vi "Rotate_Blade.vi"(7 "Activate Rotation?":bool, 8 "error in":errorcluster, 9 "Axis":cluster{"X":sgl, "Y":sgl, "Z":sgl}, 10 "angle":sgl, 11 "Scene Object In":refnum<vi>) -> (0 "error out":errorcluster, 3 "Scene Object Out":refnum<vi>)   [LabVIEW 2019]
uses:
  <vilib>/picture/3D Picture Control/NI_3D Picture Control.lvlib
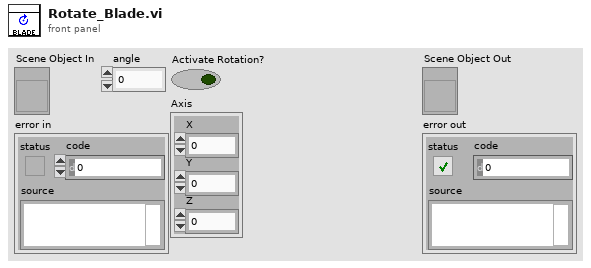
[diagram p1: front panel]
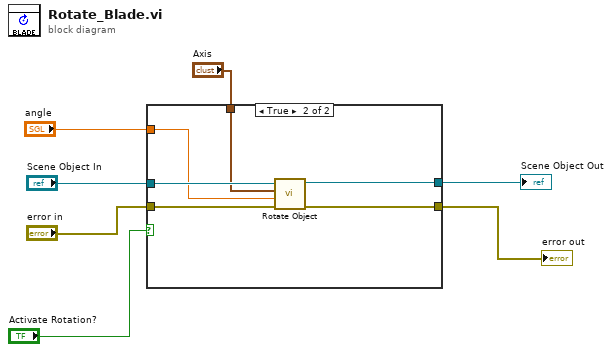
[diagram p0: block diagram]
diagram:
  n1 = case shown="True" "Activate Rotation?" {
    tunnel: [w9 w15] -> w7
    tunnel: "Scene Object In" -> [w9 w14]
    tunnel: "error in" -> [w8 w13]
    tunnel: [w8 w12] -> w4
    tunnel: "angle" -> [_ w11]
    tunnel: "Axis" -> [_ w10]
    frame False {
    }
    frame True {
      n2 = call <vilib>:"Rotate Object.vi"("error in (no error)"=w13, "Angle"=w11, "Axis"=w10, "Scene.Object In"=w14) -> ("error out"=w12:errorcluster, "Scene.Object Out"=w15:refnum<vi>)  [unwired: 6 in]
    }
  }
  "Scene Object Out" <- w7
  "error out" <- w4
